vi "visualise_aux.vi"(8 "error in (no error)":errorcluster, 11 "dataTA in":refnum<class "dataTA.lvclass">) -> (0 "error out":errorcluster, 3 "dataTA out":refnum<class "dataTA.lvclass">)   [LabVIEW 2019, in "dataTA.lvlib" / "dataTA.lvclass"]
uses:
  dataTA.lvclass
  dataTA.lvclass/dataTA.ctl
panel:
  out "max value":dbl
  out "x*y":dbl
  in  "x/y":bool
  out "Intensity Graph 2":dbl[][](graph)
  # "Pixel"
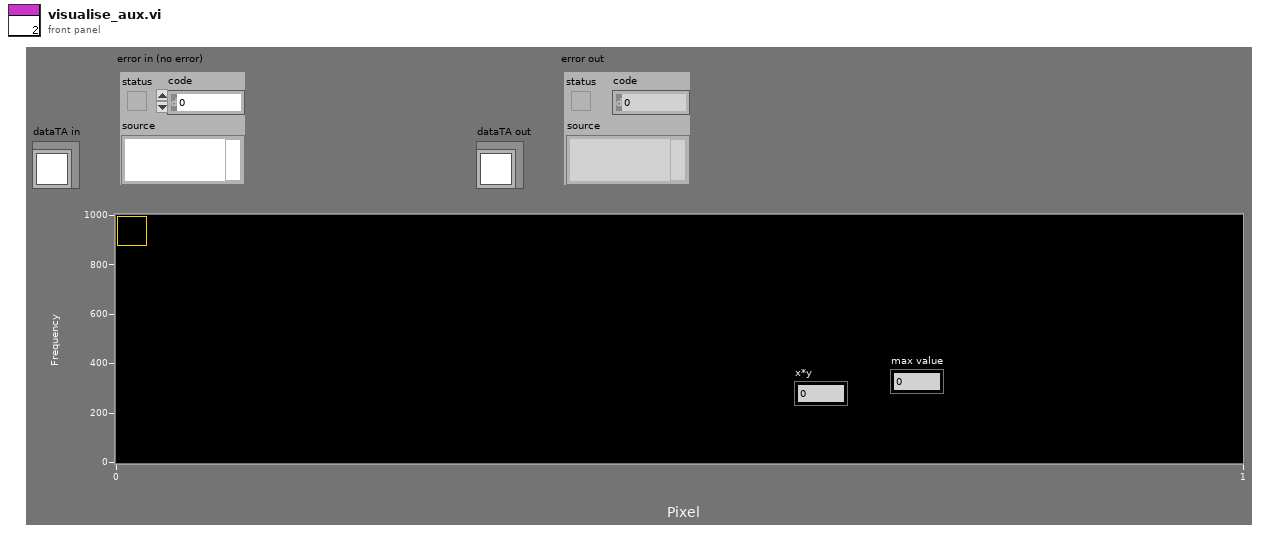
[diagram p1: front panel]
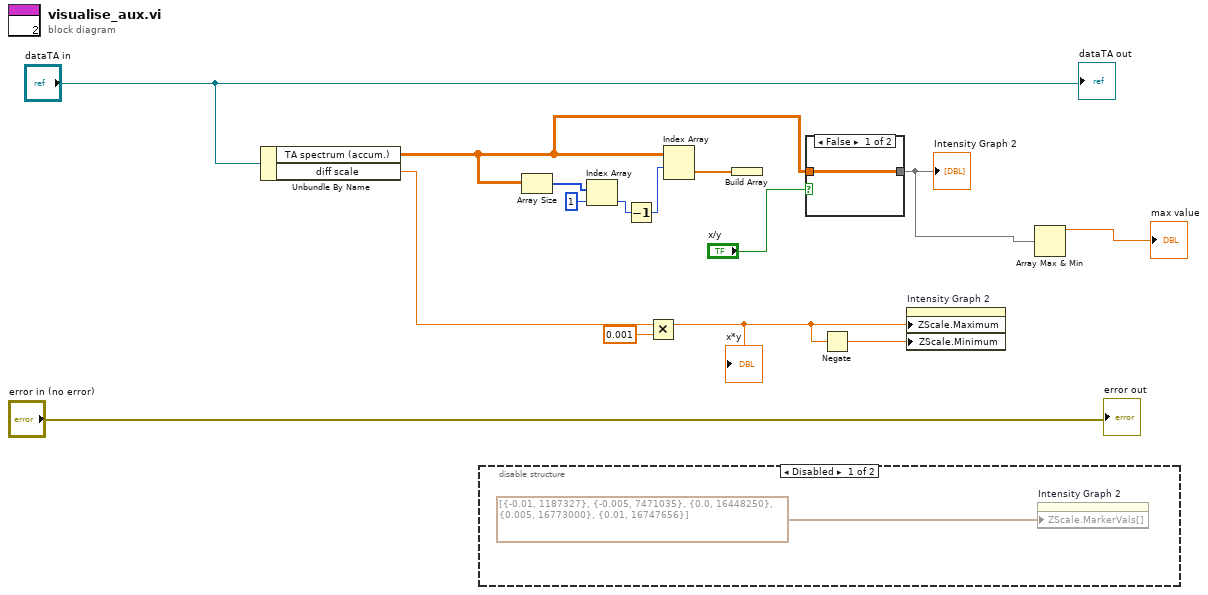
[diagram p0: block diagram]
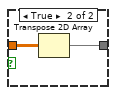
[diagram p3: hidden frame]
diagram:
  n1 = Unbundle By Name("dataTA in") -> ("TA spectrum (accum.)"=w7:dbl[][], "diff scale"=w5:dbl)
  n2 = disable-structure shown="Disabled" {
    frame Disabled {
      n3 = property on="Intensity Graph 2" class="IntGraph (strict)"("ZScale.MarkerVals[]"=cluster{dbl, u32}[] [{-0.01, 1187327}, {-0.005, 7471035}, {0.0, 16448250}, {0.005, 16773000}, {0.01, 16747656}] ("Z Scale.Marker Values[]")) -> ()  [unwired: 2 in, 2 out]
    }
    frame Enabled {
    }
  }
  n4 = Array Size(array=w7) -> (size(s)=w13:i32[])
  n5 = Index Array(array=w13, index=1) -> (element=w11:i32)
  n6 = Decrement(x=w11) -> (x-1=w10:i32)
  n7 = Multiply(x=w5, y=0.001) -> (x*y=w4:dbl)
  "x*y" <- w4
  n8 = Index Array(array=w7, index (row)=w10) -> (element=w9:dbl[])  [unwired: 1 in]
  n9 = Build Array(w9) -> ()  [unwired: 1 out]
  n10 = case shown="False" "x/y" {
    tunnel: w7 -> [w17 w19]
    tunnel: [w17 w18] -> w1
    frame False {
    }
    frame True {
      n11 = Transpose 2D Array(2D array=w19) -> (transposed array=w18:dbl[][])
    }
  }
  "Intensity Graph 2" <- w1
  n12 = Negate(x=w4) -> (-x=w6:dbl)
  n13 = property on="Intensity Graph 2" class="IntGraph (strict)"("ZScale.Maximum"=w4, "ZScale.Minimum"=w6) -> ()  [unwired: 2 in, 2 out]
  n14 = Array Max & Min(array=w1) -> (max value=→"max value":dbl)  [unwired: 3 out]
  "error out" <- "error in (no error)"
  "dataTA out" <- "dataTA in"
